vi "DHE_DRV_artif_pattern.vi"(0 "fd":i32, 7 "type":i16, 9 "params":string, 11 "error in (no error)":errorcluster) -> (4 "fd out":i32, 8 "return value":i32, 15 "error out":errorcluster)   [LabVIEW 2016]
doc: "This VI opens (Flag=1) or closes (Flag=0) the instrument shutter."
uses:
  c/lib/libarcDHE.so
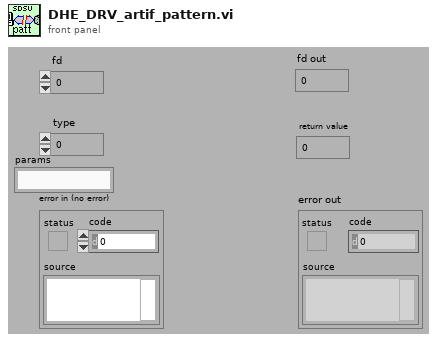
[diagram p1: front panel]
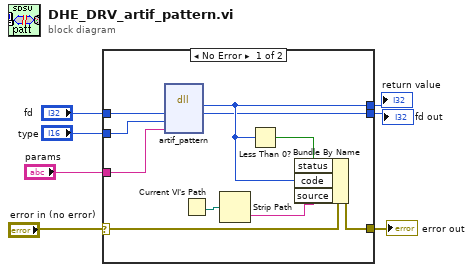
[diagram p0: block diagram]
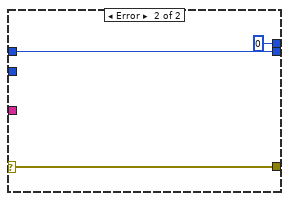
[diagram p2: hidden frame]
diagram:
  n1 = case shown="No Error" "error in (no error)" {
    selector: "error in (no error)" -> [w10 w18]
    tunnel: "fd" -> [w17 w20]
    tunnel: [w15 0] -> w6
    tunnel: [w12 w18] -> w5
    tunnel: "type" -> [w9 _]
    tunnel: [w11 w20] -> w3
    tunnel: "params" -> [w8 _]
    frame No Error {
      n2 = dll-call lib="home/simager/panview/PAN/Modules/SDSU/private/c/lib/libarcDHE.so" fn="artif_pattern" label="artif data"("fd"=w17, "type"=w9, "args"=w8) -> ("return type"=w15:i32, "fd"=w11:i32)  [unwired: 5 in, 2 out]
      n3 = Current VI's Path() -> (path=w14:path)
      n4 = Strip Path(path=w14) -> (name=w13:string)  [unwired: 1 out]
      n5 = Less Than 0?(x=w15) -> (x < 0?=w16:bool)
      n6 = Bundle By Name(cluster=w10, "status"=w16, "code"=w15, "source"=w13) -> (w12:errorcluster)
    }
    frame Error {
    }
  }
  "error out" <- w5
  "return value" <- w6
  "fd out" <- w3
